vi "DisconnectFromRobot.vi"(2 "UR Robot":refnum<k24>, 3 "error in":errorcluster) -> (1 "error out":errorcluster)   [LabVIEW 2016, in "UnderAutomation.UniversalRobots.lvlib"]
uses:
  UnderAutomation.UniversalRobots.lvlib
  C:/Users/fg/Documents/UniversalRobots.vi/LabVIEW_2024/UnderAutomation.UniversalRobots/lib/UnderAutomation.UniversalRobots.dll
  LabVIEW_2024/UnderAutomation.UniversalRobots/lib/UnderAutomation.UniversalRobots.dll
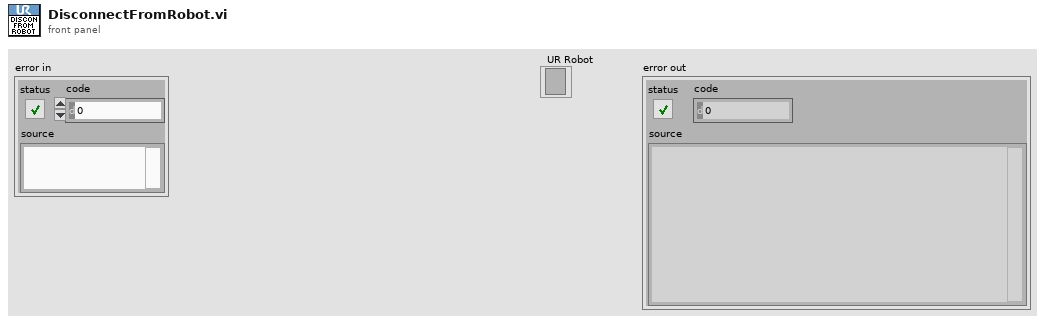
[diagram p1: front panel]
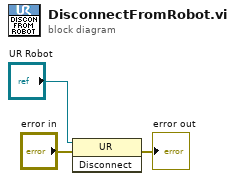
[diagram p0: block diagram]
diagram:
  n1 = invoke class="UR" method="Disconnect"(reference="UR Robot", error in="error in") -> (error out=→"error out":errorcluster)  [unwired: 1 in, 2 out]
